vi "String Indicator.vi"(10 "String Indicator":string, 11 "Dev Panel in":refnum<class "Dev Panel.lvclass">) -> (0 "error out":errorcluster)   [LabVIEW 2021, in "Dev Panel.lvclass"]
uses:
  Dev Panel.lvclass
  Dev Panel.lvclass/Dev Panel.ctl
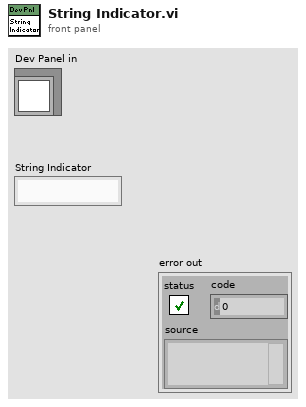
[diagram p1: front panel]
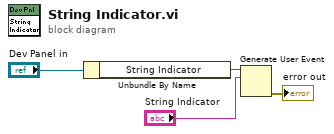
[diagram p0: block diagram]
diagram:
  n1 = Unbundle By Name("Dev Panel in") -> ("String Indicator"=w4:refnum<user-event>)
  n2 = Generate User Event(user event=w4, event data cluster="String Indicator") -> (error out=→"error out":errorcluster)  [unwired: 2 in, 1 out]
